vi "Dequeue Message.vi"(8 "error in (no error)":errorcluster caption="错误输入（无错误）", 11 "Message Queue":refnum<queue> caption="消息队列") -> (0 "error out":errorcluster caption="错误输出", 1 "Message Data":variant caption="消息数据", 2 "Message":string caption="消息", 3 "dup Message Queue":refnum<queue> caption="消息队列副本")   [LabVIEW 2013, in "Message Queue.lvlib"]
doc: "本VI从消息队列中取出消息。本VI对“消息处理循环”最后一个迭代中出错的情况实现了错误处理。\n\n无错误 - 按常规执行“元素出队列”操作。\n错误 - 检查错误代码，判断是否是可忽略的错误。如出现可忽略的错误，则按常规执行“元素出队列”操作。否则，输出该错误，并将“停止”消息加入“消息队列”。"
uses:
  Message Queue.lvlib
  Message Cluster.ctl
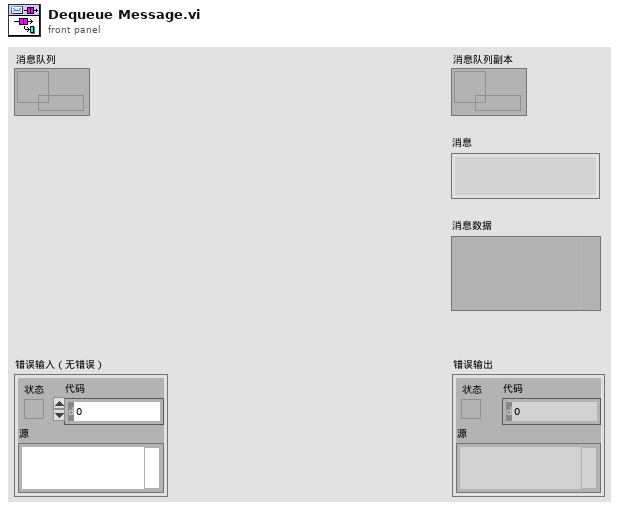
[diagram p1: front panel]
types:
  T1 = typedef "Message Queue.lvlib/Message Cluster.ctl" = cluster{"Message":string, "Message Data":variant}
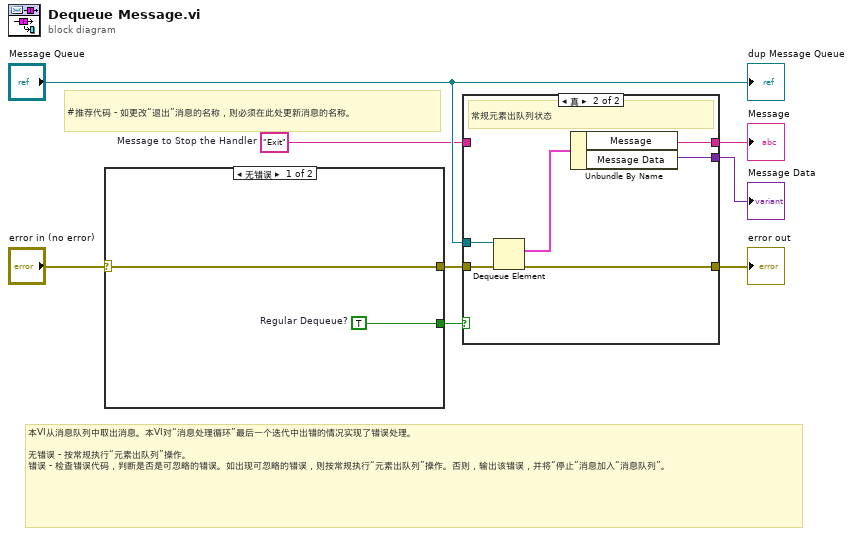
[diagram p0: block diagram]
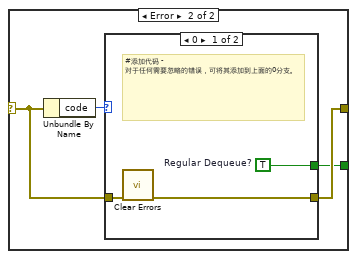
[diagram p3: hidden frame]
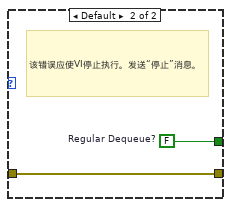
[diagram p4: hidden frame]
diagram:
  w1 = "Exit"  # Message to Stop the Handler
  # "#推荐代码 - 如更改“退出”消息的名称，则必须在此处更新消息的名称。"
  # "本VI从消息队列中取出消息。本VI对“消息处理循环”最后一个迭代中出错的情况实现了错误处理。\n\n无错误 - 按常规执行“元素出队列”操作。\n错误 - 检查错误代码，判断是否是可忽略的错误。如出现可忽略的错误，则按常规执行“元素出队列”操作。否则，输出该错误，并将“停止”消息加入“消息队列”。"
  n1 = case shown="无错误" "error in (no error)" {
    selector: "error in (no error)" -> [w10 w13]
    tunnel: [w10 w12] -> w6
    tunnel: [w9 w11] -> w5
    frame No Error {
      w9 = TRUE  # Regular Dequeue?
    }
    frame Error {
      n2 = Unbundle By Name(w13) -> ("code"=w14:i32)
      n3 = case shown="0" w14 {
        tunnel: [w17 w19] -> w12
        tunnel: w13 -> [w16 w19]
        tunnel: [w15 w18] -> w11
        frame 0 {
          w15 = TRUE  # Regular Dequeue?
          # "#添加代码 - 对于任何需要忽略的错误，可将其添加到上面的0分支。"
          n4 = call <vilib>:"Clear Errors.vi"("error in (no error)"=w16) -> ("error out"=w17:errorcluster)  [unwired: 6 in]
        }
        frame Default {
          w18 = FALSE  # Regular Dequeue?
          # "该错误应使VI停止执行。发送“停止”消息。"
        }
      }
    }
  }
  n5 = case shown="真" w5 {
    tunnel: [w21 w27] -> w7
    tunnel: w6 -> [w21 w26]
    tunnel: "Message Queue" -> [_ w25]
    tunnel: [w20 w23] -> w3
    tunnel: [_ w22] -> w2
    tunnel: w1 -> [w20 _]
    frame False {
      # "错误"
    }
    frame True {
      # "常规元素出队列状态"
      n6 = Dequeue Element(queue=w25, error in (no error)=w26) -> (element=w24:T1, error out=w27:errorcluster)  [unwired: 1 in, 2 out]
      n7 = Unbundle By Name(w24) -> ("Message"=w23:string, "Message Data"=w22:variant)
    }
  }
  "error out" <- w7
  "Message" <- w3
  "Message Data" <- w2
  "dup Message Queue" <- "Message Queue"
